vi "sub_check_logged_in.vi"(8 "error in (no error)":errorcluster, 11 "daq.io type in":T1={"daq.io ref"=refnum, "daq.io API Base"="http://dashboard.daq.io/api/v1", "Device Type Key"="", "Device Key"="", "Account ID"=""}) -> (0 "error out":errorcluster, 2 "logged in?":bool, 3 "daq.io type out":T1={"daq.io ref"=refnum, "daq.io API Base"="http://dashboard.daq.io/api/v1", "Device Type Key"="", "Device Key"="", "Account ID"=""})   [LabVIEW 2013, in "daqio minimal.lvlib"]
doc: "This VI checks whether the user is logged in correctly. It will return \"false\" when the user cannot log in. It will return the user's account ID if connected and logged in. If the credentials are correct and this VI returns \"false\" check the Internet connection and cloud connectivity."
uses:
  daqio minimal.lvlib
  _typedefs/daqio-Type.ctl
  <vilib>/httpClient/ClientHandle.ctl
  <vilib>/Easy HTTP Client/Easy HTTP.lvlib
  <vilib>/httpClient/LabVIEWHTTPClient.lvlib
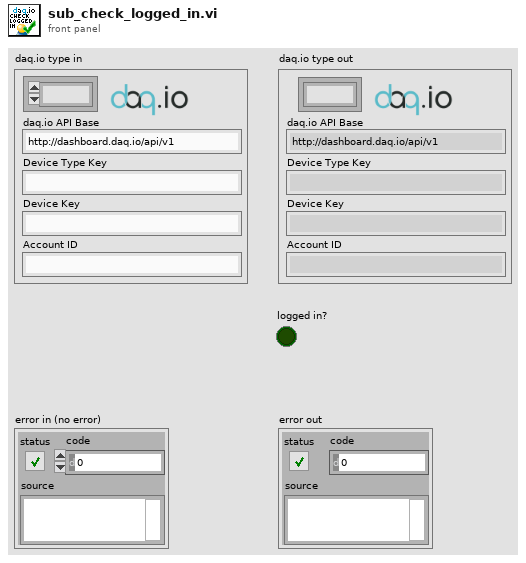
[diagram p1: front panel]
types:
  T1 = typedef "daqio minimal.lvlib/daqio-Type.ctl" = cluster{"daq.io ref":T2, "daq.io API Base":string, "Device Type Key":string, "Device Key":string, "Account ID":string}
  T2 = typedef "LabVIEWHTTPClient.lvlib/ClientHandle.ctl" = refnum<k1>
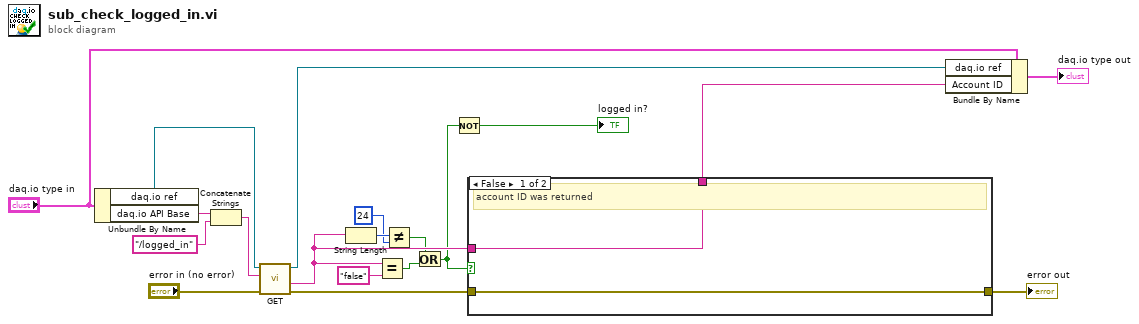
[diagram p0: block diagram]
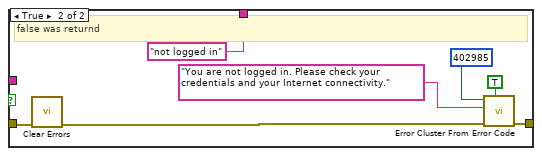
[diagram p2: hidden frame]
diagram:
  n1 = Unbundle By Name("daq.io type in") -> ("daq.io ref"=w14:T2, "daq.io API Base"=w12:string)
  n2 = Concatenate Strings(w12, "/logged_in" ("string")) -> (w18:string)
  n3 = call <vilib>:"GET.vi"("error in (no error)"="error in (no error)", "url"=w18, "client handle"=w14) -> ("error out"=w10:errorcluster, "body"=w6:string, "client handle out"=w11:T2)  [unwired: 4 in, 2 out]
  n4 = String Length(string=w6) -> (length=w5:i32)
  n5 = Equal?(x=w6, y="false") -> (x = y?=w3:bool)
  n6 = Not Equal?(x=w5, y=24) -> (x != y?=w2:bool)
  n7 = Or(x=w2, y=w3) -> (x .or. y?=w1:bool)
  n8 = Not(x=w1) -> (.not. x?=→"logged in?":bool)
  n9 = case shown="False" w1 {
    tunnel: w10 -> [w21 w24]
    tunnel: [w21 w26] -> w13
    tunnel: w6 -> [w20 _]
    tunnel: [w20 "not logged in" ("body")] -> w9
    frame False {
      # "account ID was returned"
    }
    frame True {
      # "false was returnd"
      n10 = call <vilib>:"Clear Errors.vi"("error in (no error)"=w24) -> ("error out"=w23:errorcluster)  [unwired: 6 in]
      n11 = call <vilib>:"Error Cluster From Error Code.vi"("show call chain? (False)"=TRUE, "error in (no error)"=w23, "error message (\"\")"="You are not logged in. Please check your credentials and your Internet connectivity." ("error message (\"\")"), "error code (0)"=402985) -> ("error out"=w26:errorcluster)  [unwired: 5 in]
    }
  }
  "error out" <- w13
  n12 = Bundle By Name(cluster="daq.io type in", "daq.io ref"=w11, "Account ID"=w9) -> (→"daq.io type out":T1)
